vi "joystickVSS.vi"() -> ()   [LabVIEW 2017]
uses:
  Core/AI Robot.ctl
  Intel/Functions Enum.ctl
  Intel/AttackerStates.ctl
  Path Planning/RRT/PathDests.ctl
  Path Planning/RRT/PathDest.ctl
  <vilib>/Instr/_visa.llb/VISA Configure Serial Port (Instr).vi
panel:
  in  "k":dbl=0.1 format="%#_13g"
  out "Array":T1[](array[typedef])
  in  "IDs":u32[](array[numeric])
  out "Numeric 2":dbl
  out "String":string
  out "return count":u32
  in  "stop":bool
  out "string":string
  out "error out":errorcluster
  in  "termination char\n(0xA = '\\n' = LF)":u8=10 format="%.0x"
  in  "VISA resource name":refnum<visa-resource-name>
  in  "Serial Settings":T6={"baud rate"=9600, "data bits"=8, "parity"=enum."None", "stop bits"=10, "flow control"=0} {"flow control" items=["None"=0, "XON/XOFF"=1, "RTS/CTS"=2, "DTR/DSR"=4]; "stop bits" items=["1.0"=10, "1.5"=15, "2.0"=20]; "data bits" min=5 max=8 step=1; "baud rate" items=["75"=75, "110"=110, "134"=134, "150"=150, "300"=300, "600"=600, "1200"=1200, "1800"=1800, "2400"=2400, "4800"=4800, "7200"=7200, "9600"=9600, "14400"=14400, "19200"=19200, "28800"=28800, "38400"=38400, "56000"=56000, "57600"=57600, "115200"=115200, "128000"=128000, "230400"=230400]}
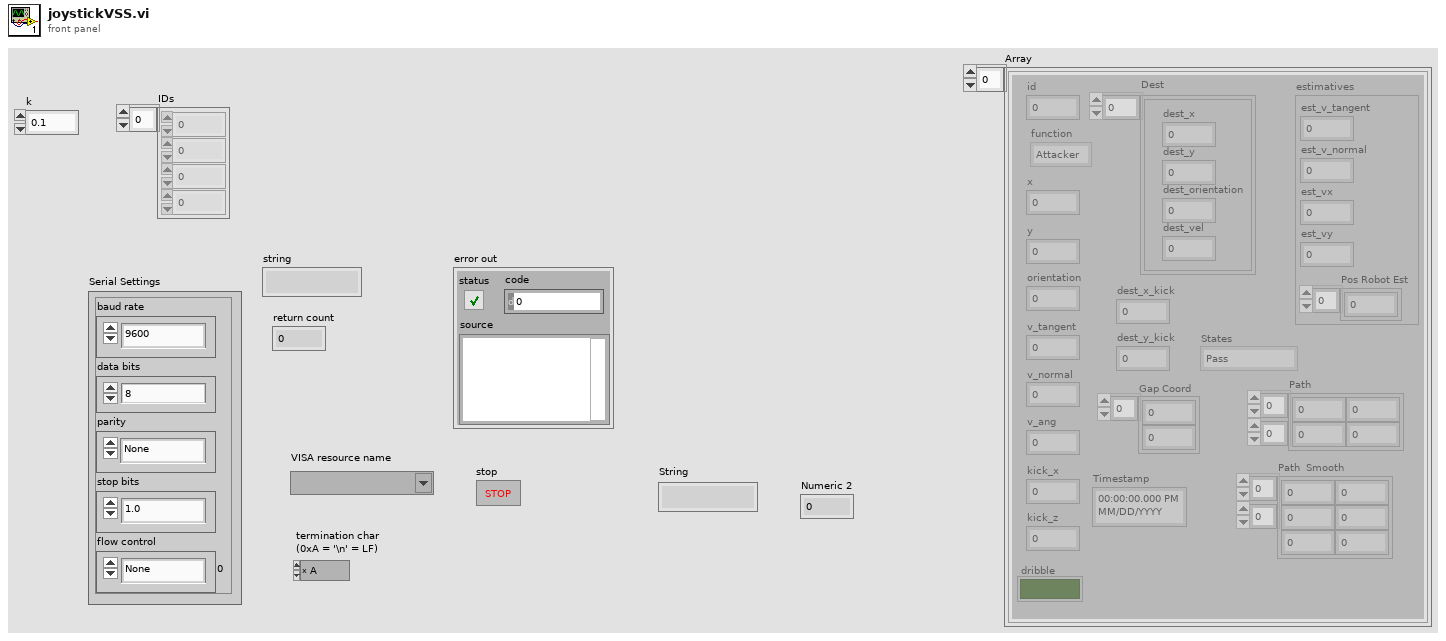
[diagram p1: front panel]
types:
  T1 = typedef "AI Robot.ctl" = cluster{"id":u32, "function":T2, "x":dbl, "y":dbl, "orientation":dbl, "v_tangent":dbl, "v_normal":dbl, "v_ang":dbl, "kick_x":dbl, "kick_z":dbl, "dribble":bool, "Timestamp":timestamp, "estimatives":cluster{"est_v_tangent":dbl, "est_v_normal":dbl, "est_vx":dbl, "est_vy":dbl, "Pos Robot Est":dbl[]}, "dest_x_kick":dbl, "dest_y_kick":dbl, "Gap Coord":dbl[], "States":T3, "Path ":dbl[][], "Path  Smooth":dbl[][], "Dest":T4}
  T2 = typedef "Functions Enum.ctl" = enum16{"Attacker", "Goalie", "Defender", "Striker", "Goto 0", "Dummy", "Kicker", "ZigZag"}
  T3 = typedef "AttackerStates.ctl" = enum16{"Pass", "GoToTangent", "BallGetting", "GoToKick", "Rotate anti-clockwise", "Rotate Clockwise", ""}
  T4 = typedef "PathDests.ctl" = T5[]
  T5 = typedef "PathDest.ctl" = cluster{"dest_x":dbl, "dest_y":dbl, "dest_orientation":dbl, "dest_vel":dbl}
  T6 = cluster{"baud rate":u32, "data bits":u16, "parity":enum16{"None", "Odd", "Even", "Mark", "Space"}, "stop bits":u16, "flow control":u16}
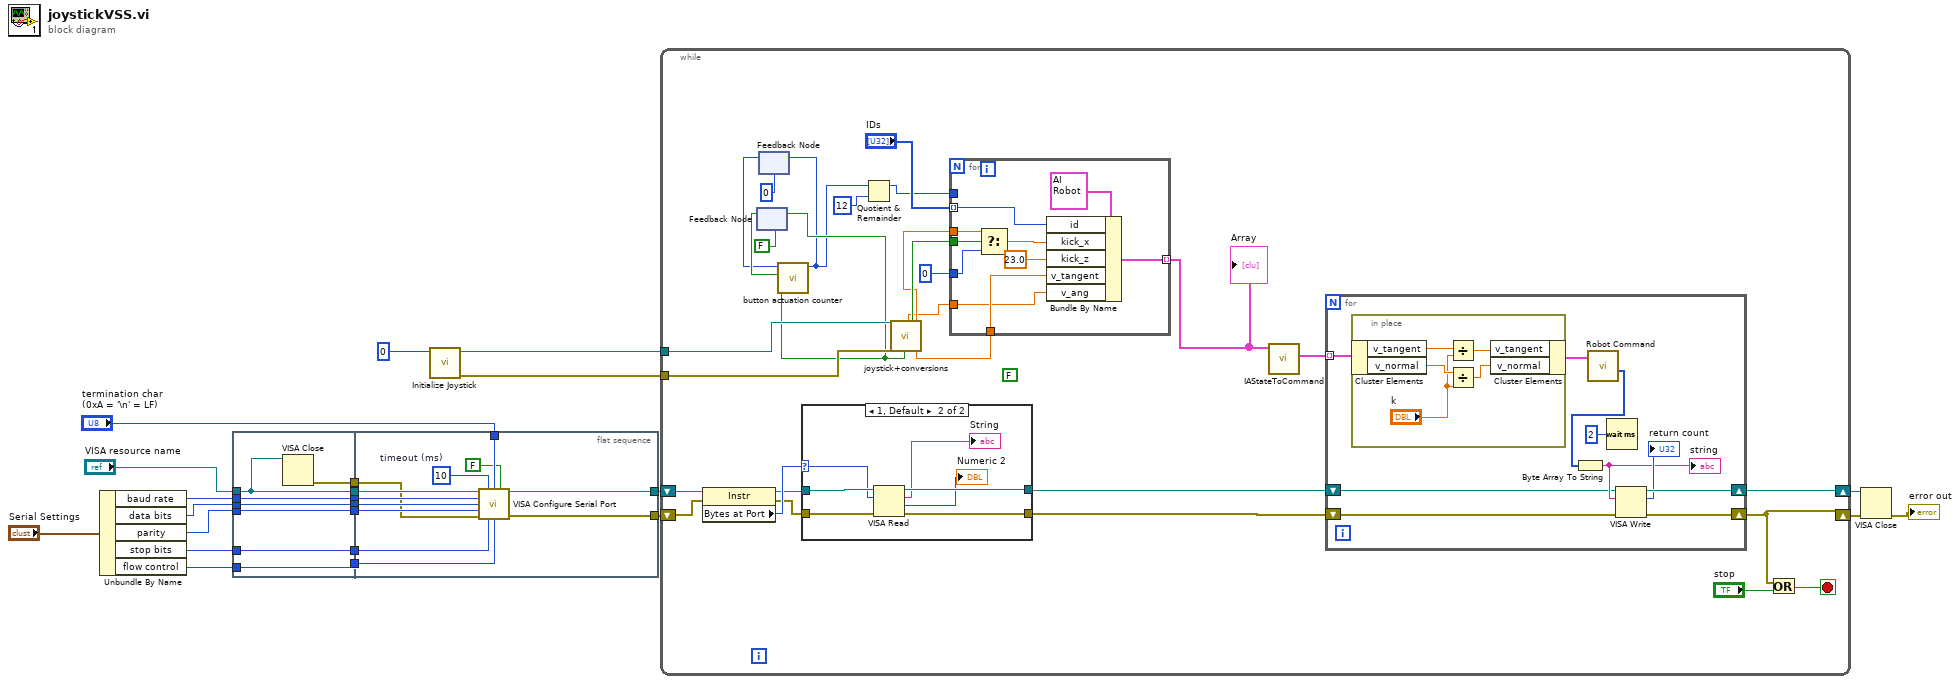
[diagram p0: block diagram]
diagram:
  n1 = Unbundle By Name("Serial Settings") -> ("baud rate"=w22:u32, "data bits"=w21:u16, "parity"=w20:enum16{"None", "Odd", "Even", "Mark", "Space"}, "stop bits"=w19:u16, "flow control"=w18:u16)
  n2 = flat-sequence {
    tunnel: "VISA resource name" -> [w25]
    tunnel: w18 -> [w26]
    tunnel: w19 -> [w27]
    tunnel: w20 -> [w28]
    tunnel: w21 -> [w29]
    tunnel: w22 -> [w30]
    tunnel: [w30] -> w7
    tunnel: [w29] -> w6
    tunnel: [w28] -> w5
    tunnel: [w27] -> w4
    tunnel: [w26] -> w3
    tunnel: [w25] -> w2
    tunnel: [w24] -> w1
    tunnel: "termination char\n(0xA = '\\n' = LF)" -> [w36]
    tunnel: [w34] -> w15
    tunnel: [w33] -> w13
    tunnel: w7 -> [w42]
    tunnel: w6 -> [w41]
    tunnel: w5 -> [w40]
    tunnel: w4 -> [w39]
    tunnel: w3 -> [w38]
    tunnel: w2 -> [w37]
    tunnel: w1 -> [w31]
    frame #0 {
      n3 = VISA Close(VISA resource name=w25) -> (error out=w24:errorcluster)  [unwired: 1 in]
    }
    frame #1 {
      w32 = u32 10  # timeout (ms)
      n4 = call-poly "VISA Configure Serial Port"("VISA resource name"=w37, "timeout (10sec)"=w32, "termination char\n(0xA = '\\n' = LF)"=w36, "Enable Termination\nChar (T)"=FALSE ("Enable Termination\nChar (T)"), "baud rate (9600)"=w42, "data bits (8)"=w41, "parity (0:none)"=w40, "error in (no error)"=w31, "stop bits (10: 1 bit)"=w39, "flow control (0:none)"=w38) -> ("VISA resource name out"=w34:refnum<visa-resource-name>, "error out"=w33:errorcluster)  [unwired: 4 in]
    }
  }
  n5 = call <vilib>:"Initialize Joystick.vi"("device index"=0) -> ("error out"=w8:errorcluster, "device ID"=w9:refnum<k1>)  [unwired: 9 in]
  n6 = while {
    shift-right: [w71] -> w14
    shift-left: w15 -> [w55]
    shift-right: [w69] -> w12
    shift-left: w13 -> [w54]
    tunnel: w9 -> [w68]
    tunnel: w8 -> [w67]
    stop <- w70 stop-if-true
    (unwired) FALSE
    n7 = property class="Instr"(reference=w55, error in=w54) -> (reference out=w51:refnum<visa-resource-name>, error out=w52:errorcluster, "Bytes at Port"=w53:u32)
    n8 = feedback #1(FALSE) -> (w64:bool)
    n9 = feedback #2(0) -> (w62:i32)
    n10 = case shown="1, Default" w53 {
      selector: w53 -> [_ w99]
      tunnel: w52 -> [w97 w105]
      tunnel: [w97 w104] -> w57
      tunnel: w51 -> [w98 w103]
      tunnel: [w98 w102] -> w56
      frame 0 {
      }
      frame 1, Default {
        n11 = VISA Read(VISA resource name=w103, byte count=w99, error in (no error)=w105) -> (VISA resource name out=w102:refnum<visa-resource-name>, read buffer=→"String":string, return count=→"Numeric 2":u32, error out=w104:errorcluster)
      }
    }
    n12 = call "joystick+conversions.vi"("Refnum in"=w68, "error in (no error)"=w67) -> ("B pressed"=w65:bool, "v_radial"=w48:dbl, "A pressed"=w59:bool, "chute"=w58:dbl, "v_normal"=w49:dbl)  [unwired: 9 in, 12 out]
    n13 = feedback-in #1(w65) -> ()
    n14 = call "button actuation counter.vi"("old count"=w62, "was button pressed ?"=w64, "button pressed now"=w65) -> ("new count"=w50:i32)  [unwired: 7 in]
    n15 = feedback-in #2(w50) -> ()
    n16 = Quotient & Remainder(x=w50, y=12) -> (x-y*floor(x/y)=w44:i32)  [unwired: 1 out]
    n17 = for {
      tunnel: 0 ("f") -> [w81]
      tunnel: w59 -> [w80]
      tunnel: w58 -> [w79]
      tunnel: "IDs" -> [w78] mode=indexing
      tunnel: w49 -> [w75]
      tunnel: w48 -> [w74]
      tunnel: w44 -> [_]
      tunnel: [w73] -> w43 mode=indexing
      n18 = Select(t=w79, s=w80, f=w81) -> (s? t:f=w77:dbl)
      n19 = Bundle By Name(cluster=T1 {"id"=0, "function"=enum."Attacker", "x"=0.0, "y"=0.0, "orientation"=0.0, "v_tangent"=0.0, "v_normal"=0.0, "v_ang"=0.0, "kick_x"=0.0, "kick_z"=0.0, "dribble"=FALSE, "Timestamp"=timestamp(0 s since 1904-01-01), "estimatives"={"est_v_tangent"=0.0, "est_v_normal"=0.0, "est_vx"=0.0, "est_vy"=0.0, "Pos Robot Est"=[]}, "dest_x_kick"=0.0, "dest_y_kick"=0.0, "Gap Coord"=[], "States"=enum."Pass", "Path "=[], "Path  Smooth"=[], "Dest"=[]} ("element"), "id"=w78, "kick_x"=w77, "kick_z"=sgl 23.0 ("kickspeedx"), "v_tangent"=w75, "v_ang"=w74) -> (w73:T1)
    }
    "Array" <- w43
    n20 = call "IAStateToCommand.vi"("our_robots"=w43) -> ("robots out"=w46:T1[])  [unwired: 9 in, 1 out]
    n21 = for {
      shift-right: [w89] -> w69
      shift-left: w57 -> [w86]
      shift-right: [w91] -> w71
      shift-left: w56 -> [w85]
      tunnel: w46 -> [w84] mode=indexing
      n22 = in-place {
        n23 = in-place-cluster #3(w84) -> ("v_tangent"=w96:dbl, "v_normal"=w94:dbl)
        n24 = Divide(x=w96, y="k") -> (x/y=w95:dbl)
        n25 = Divide(x=w94, y="k") -> (x/y=w93:dbl)
        n26 = in-place-cluster #3("v_tangent"=w95, "v_normal"=w93) -> (w83:T1)
      }
      n27 = call "Robot Command.vi"("Robot"=w83) -> ("Array"=w82:u8[])  [unwired: 10 in]
      n28 = Byte Array To String(unsigned byte array=w82) -> (string=w87:string)
      "string" <- w87
      n29 = Wait (ms)(milliseconds to wait=u32 2) -> ()  [unwired: 1 out]
      n30 = VISA Write(VISA resource name=w85, write buffer=w87, error in (no error)=w86) -> (VISA resource name out=w91:refnum<visa-resource-name>, return count=→"return count":u32, error out=w89:errorcluster)
    }
    n31 = Or(x=w69, y="stop") -> (x .or. y?=w70:bool)
  }
  n32 = VISA Close(VISA resource name=w14, error in (no error)=w12) -> (error out=→"error out":errorcluster)
